vi "tx streamer send.vi"(0 "h":u64, 1 "timeout":dbl, 5 "buffs":csg[](array[numeric]), 9 "md":u64, 11 "error in (no error)":errorcluster, 12 "items_sent":u64) -> (4 "h 2":u64, 6 "buffs out":csg[](array[numeric]), 8 "function return":u32(ring), 10 "md out":u64, 14 "items_sent out":u64, 15 "error out":errorcluster)   [LabVIEW 2024, in "uhd.lvlib"]
doc: "UHD_API uhd_error uhd_tx_streamer_send(uhd_tx_streamer_handle h,\n const void** buffs,\n size_t samps_per_buff,\n uhd_tx_metadata_handle* md,\n double timeout,\n size_t* items_sent);"
uses:
  uhd.lvlib
  uhd.so
panel:
  in  "samps_per_buff":u64
  in  "buffs":u32
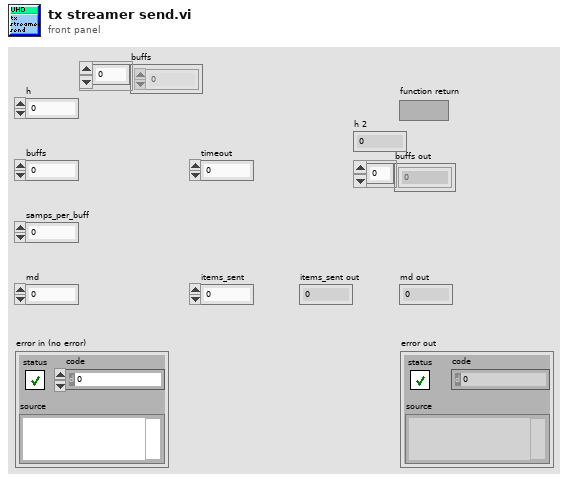
[diagram p1: front panel]
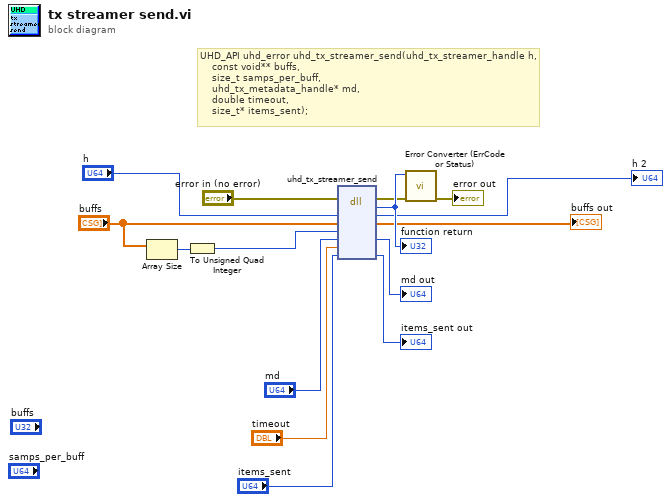
[diagram p0: block diagram]
diagram:
  # "UHD_API uhd_error uhd_tx_streamer_send(uhd_tx_streamer_handle h,\n    const void** buffs,\n    size_t samps_per_buff,\n    uhd_tx_metadata_handle* md,\n    double timeout,\n    size_t* items_sent);"
  n1 = Array Size(array="buffs") -> (size(s)=w4:i32)
  n2 = To Unsigned Quad Integer(1:w4) -> (0:w2:u64)
  n3 = dll-call lib="uhd.*" fn="uhd_tx_streamer_send"(error in="error in (no error)", "h"="h", "buffs"="buffs", "samps_per_buff"=w2, "md"="md", "timeout"="timeout", "items_sent"="items_sent") -> (error out=w7:errorcluster, "return type"=w15:u32, "h"=→"h 2":u64, "buffs"=→"buffs out":csg[], "md"=→"md out":u64, "items_sent"=→"items_sent out":u64)  [unwired: 4 in, 1 out]
  "function return" <- w15
  n4 = call "Error Converter (ErrCode or Status).vi"("error in (no error)"=w7, "error code"=w15) -> ("error out"=→"error out":errorcluster)  [unwired: 9 in]
